vi "TestStub1LoadContent.vi"() -> ()   [LabVIEW 2014]
uses:
  SubVIs/Classes/Document/SubClasses/Spreadsheet/Spreadsheet_class/Cell.ctl
  SubVIs/Classes/Document/SubClasses/Spreadsheet/Spreadsheet_class/Spreadsheet.lvclass
panel:
  out "length":i32
  out "ReturnedData 2":string[][](array[string])
  in  "Cell":T1
  out "ReturnedData":string[][](array[string])
  out "error out":errorcluster
  out "XML":string
  in  "error in (no error)":errorcluster
  in  "Path":path=path "C:/Users/Steve Watts/Desktop/NI Stuff/OpenDocument/Microsoft Open document xl saved file for steve.ods"
  # "(eg A5..C5)"
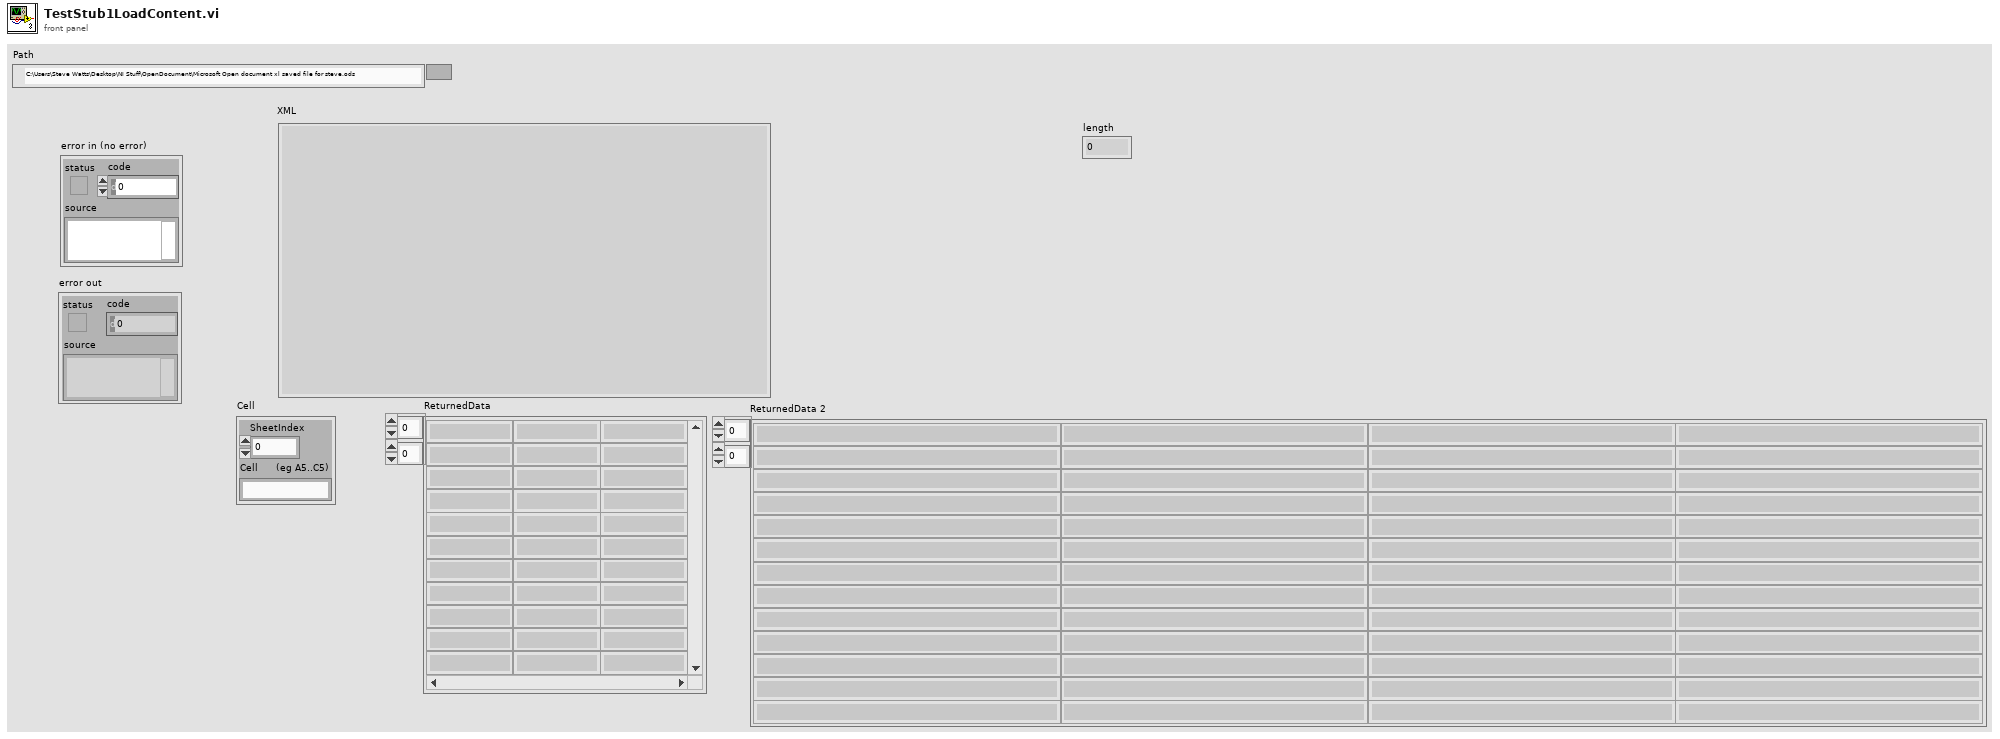
[diagram p1: front panel]
types:
  T1 = typedef "Cell.ctl" = cluster{"SheetIndex":u8, "Cell":string}
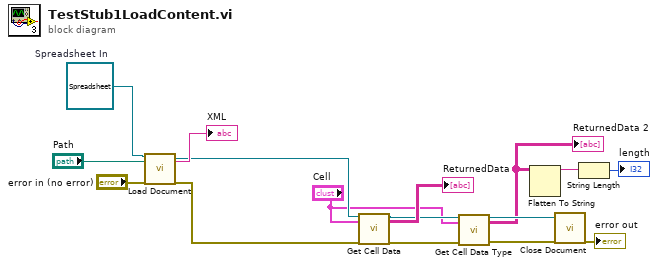
[diagram p0: block diagram]
diagram:
  w16 = refnum<class "Spreadsheet.lvclass"> refnum  # Spreadsheet In
  n1 = call-dynamic "Load Document.vi"("Spreadsheet In"=w16, "Path"="Path", "error in (no error)"="error in (no error)") -> ("Spreadsheet Out"=w9:refnum<class "Spreadsheet.lvclass">, "xml"=→"XML":string, "error out"=w8:errorcluster)  [unwired: 14 in]
  n2 = call-dynamic "Get Cell Data.vi"("object in"=w9, "Cell"="Cell", "error in (no error)"=w8) -> ("object out"=w5:refnum<class "Spreadsheet.lvclass">, "ReturnedData"=→"ReturnedData":string[][], "error out"=w6:errorcluster)  [unwired: 14 in]
  n3 = call-dynamic "Get Cell Data Type.vi"("object in"=w5, "Cell"="Cell", "error in (no error)"=w6) -> ("object out"=w11:refnum<class "Spreadsheet.lvclass">, "ReturnedData"=w3:string[][], "error out"=w10:errorcluster)  [unwired: 14 in]
  "ReturnedData 2" <- w3
  n4 = Flatten To String(anything=w3) -> (data string=w2:string)  [unwired: 3 in, 2 out]
  n5 = call-dynamic "Close Document.vi"("object in"=w11, "error in (no error)"=w10) -> ("error out"=→"error out":errorcluster)  [unwired: 16 in, 1 out]
  n6 = String Length(string=w2) -> (length=→"length":i32)
